vi "crc32.helper.vi"(9 "CRC Buffer in":u32, 10 "Data":u8, 11 "Array in":u32[](array[numeric])) -> (2 "Numeric":u32, 3 "CRC Buffer out":u32)   [LabVIEW 2020, in "fpganow.common.fpga.lvlib"]
uses:
  fpganow.common.fpga.lvlib
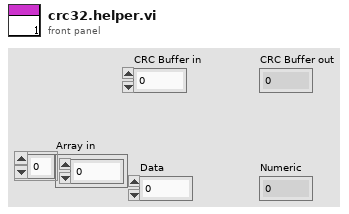
[diagram p1: front panel]
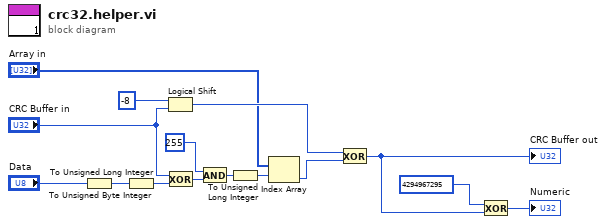
[diagram p0: block diagram]
diagram:
  n1 = To Unsigned Byte Integer(number="Data") -> (unsigned 8bit integer=w4:u8)
  n2 = To Unsigned Long Integer(number=w4) -> (unsigned 32bit integer=w10:u32)
  n3 = Logical Shift(y=-8, x="CRC Buffer in") -> (x << y=w5:u32)
  n4 = Exclusive Or(1:w10, 2:"CRC Buffer in") -> (0:w11:u32)
  n5 = And(x=u32 255, y=w11) -> (x .and. y?=w9:u32)
  n6 = To Unsigned Long Integer(number=w9) -> (unsigned 32bit integer=w7:u32)
  n7 = Index Array(array="Array in", index=w7) -> (element=w6:u32)
  n8 = Exclusive Or(1:w6, 2:w5) -> (0:w14:u32)
  "CRC Buffer out" <- w14
  n9 = Exclusive Or(1:w14, 2:u32 4294967295 ("x")) -> (0:→"Numeric":u32)
